vi "Apply Angle.vi"(8 "error in (no error)":errorcluster, 10 "ccw servo angle (rad)":dbl, 11 "servo motor in":refnum<class "NI_Robotics_Starter Kit Servo Motor_1.0.lvclass">) -> (0 "error out":errorcluster, 3 "servo motor out":refnum<class "NI_Robotics_Starter Kit Servo Motor_1.0.lvclass">)   [LabVIEW 2017, in "NI_Robotics_Starter Kit Servo Motor_1.0.lvclass"]
uses:
  <vilib>/robotics/Starter Kit/Servo Motor 1.0/NI_Robotics_Starter Kit Servo Motor_1.0.lvclass
  <vilib>/robotics/Starter Kit/Servo Motor 1.0/NI_Robotics_Starter Kit Servo Motor_1.0.lvclass/NI_Robotics_Starter Kit Servo Motor_1.0.ctl
  <instrlib>/Parallax Standard Servo/HAIOL/Parallax Standard Servo.lvclass
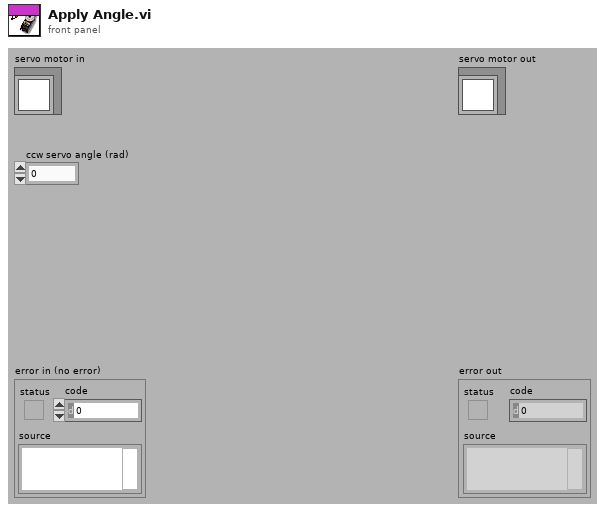
[diagram p1: front panel]
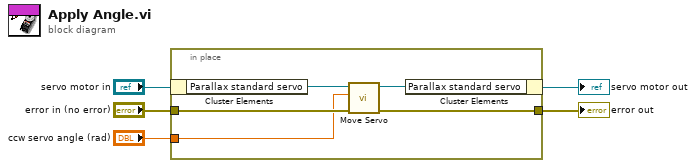
[diagram p0: block diagram]
diagram:
  n1 = in-place {
    in-place-border: "error in (no error)" -> [w8]
    in-place-border: [w7] -> w2
    in-place-border: "ccw servo angle (rad)" -> [w6]
    n2 = in-place-cluster #1("servo motor in") -> ("Parallax standard servo"=w10:refnum<class "Parallax Standard Servo.lvclass">)
    n3 = call-dynamic "Move Servo.vi"("error in (no error)"=w8, "CCW Position (0.0 rad)"=w6, "Parallax Standard Servo in"=w10) -> ("error out"=w7:errorcluster, "Parallax Standard Servo out"=w9:refnum<class "Parallax Standard Servo.lvclass">)  [unwired: 7 in]
    n4 = in-place-cluster #1("Parallax standard servo"=w9) -> (→"servo motor out":refnum<class "NI_Robotics_Starter Kit Servo Motor_1.0.lvclass">)
  }
  "error out" <- w2
